vi "SET FACTORY PATTERN.vi"(11 "Funcion":string) -> (3 "Class":string[](array[string]))   [LabVIEW 2020]
uses:
  Libraries/FGen/GeneradorAmplificado/GeneradorAmplificado.lvclass
  C:/Users/salma/IVSalma2P_2/Libraries/FGen/Generador/Generador.lvclass
  Libraries/FGen/Generador/Generador.lvclass
  C:/Users/salma/IVSalma2P_2/Libraries/FGen/GeneradorAmplificado/GeneradorAmplificado.lvclass
panel:
  out "Class":refnum<class "Generador.lvclass">
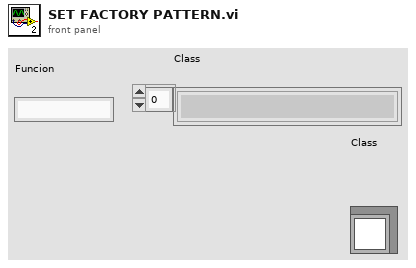
[diagram p1: front panel]
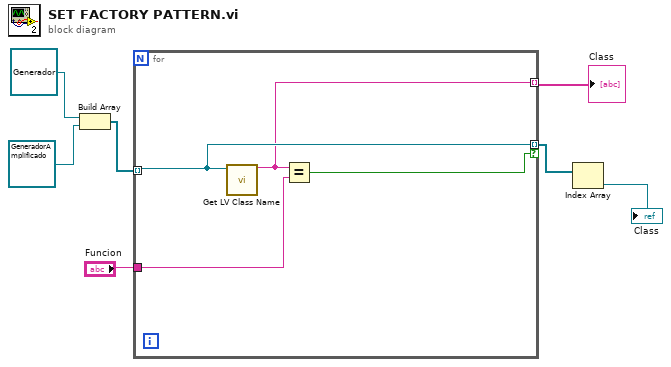
[diagram p0: block diagram]
diagram:
  n1 = Build Array(refnum<class "Generador.lvclass"> refnum ("FGen.lvlib:Generator"), refnum<class "GeneradorAmplificado.lvclass"> refnum ("FGen.lvlib:GeneradorAmplificado.lvclass")) -> (w5:refnum<class "Generador.lvclass">[])
  n2 = for {
    tunnel: w5 -> [w11] mode=indexing
    tunnel: [w11] -> w2 mode=indexing if=w9
    tunnel: "Funcion" -> [w10]
    tunnel: [w8] -> w3 mode=indexing
    n3 = call <vilib>:"Get LV Class Name.vi"("object"=w11) -> ("class name"=w8:string)  [unwired: 9 in, 1 out]
    n4 = Equal?(x=w8, y=w10) -> (x = y?=w9:bool)
  }
  "Class" <- w3
  n5 = Index Array(array=w2) -> (element=→"Class":refnum<class "Generador.lvclass">)  [unwired: 1 in]
